vi "数据库查询.vi"() -> ()   [LabVIEW 2018]
uses:
  NPOI/net40/yt_ExcelLibrary.dll
  <vilib>/addons/database/Connection.llb/DB Tools Open Connec (String).vi
  <vilib>/addons/database/NI_Database_API.lvlib
  <vilib>/addons/_office/NI_ReportGenerationToolkit.lvlib
  <vilib>/Utility/NIReport.llb/Excel/NI_Excel.lvclass
  <vilib>/addons/_office/_exclsub.llb/font.ctl
  <vilib>/ptbypt/NI_PtbyPt.lvlib
  FreeMem.dll
  <vilib>/Utility/NIReport.llb/NI_report.lvclass
  <vilib>/Utility/NIReport.llb/Report Type.ctl
  <vilib>/Utility/NIReport.llb/NI_ReportGenerationCore.lvlib
  <vilib>/addons/_office/excel.llb/Excel Easy Table (str).vi
panel:
  out "错误输出":errorcluster
  out "数字(0-1)":dbl
  out "Elapsed Time (s)":dbl caption="已用时间(s)"
  out "2天时间到释放资源":bool caption="结束"
  in  "Main Tab":enum32{""}(tab)
  in  "时间范围OFF":bool
  in  "结束日期":timestamp
  in  "起始日期":timestamp
  in  "总成码OFF":bool
  in  "总成码":string
  in  "二维码OFF":bool
  in  "二维码":string
  in  "数据类型":u16(ring) items=["ALL", "Online", "Offline", "Rework"]
  in  "产品状态":u16(ring) items=["ALL", "OK", "NG"]
  in  "导出":bool
  in  "退出":bool
  in  "查询":bool
  in  "另存为":bool
  out "查询状态":string
  out "查询结果":i32(listbox)
  # "2020-04-14_17:08"
  # "历史数据查询"
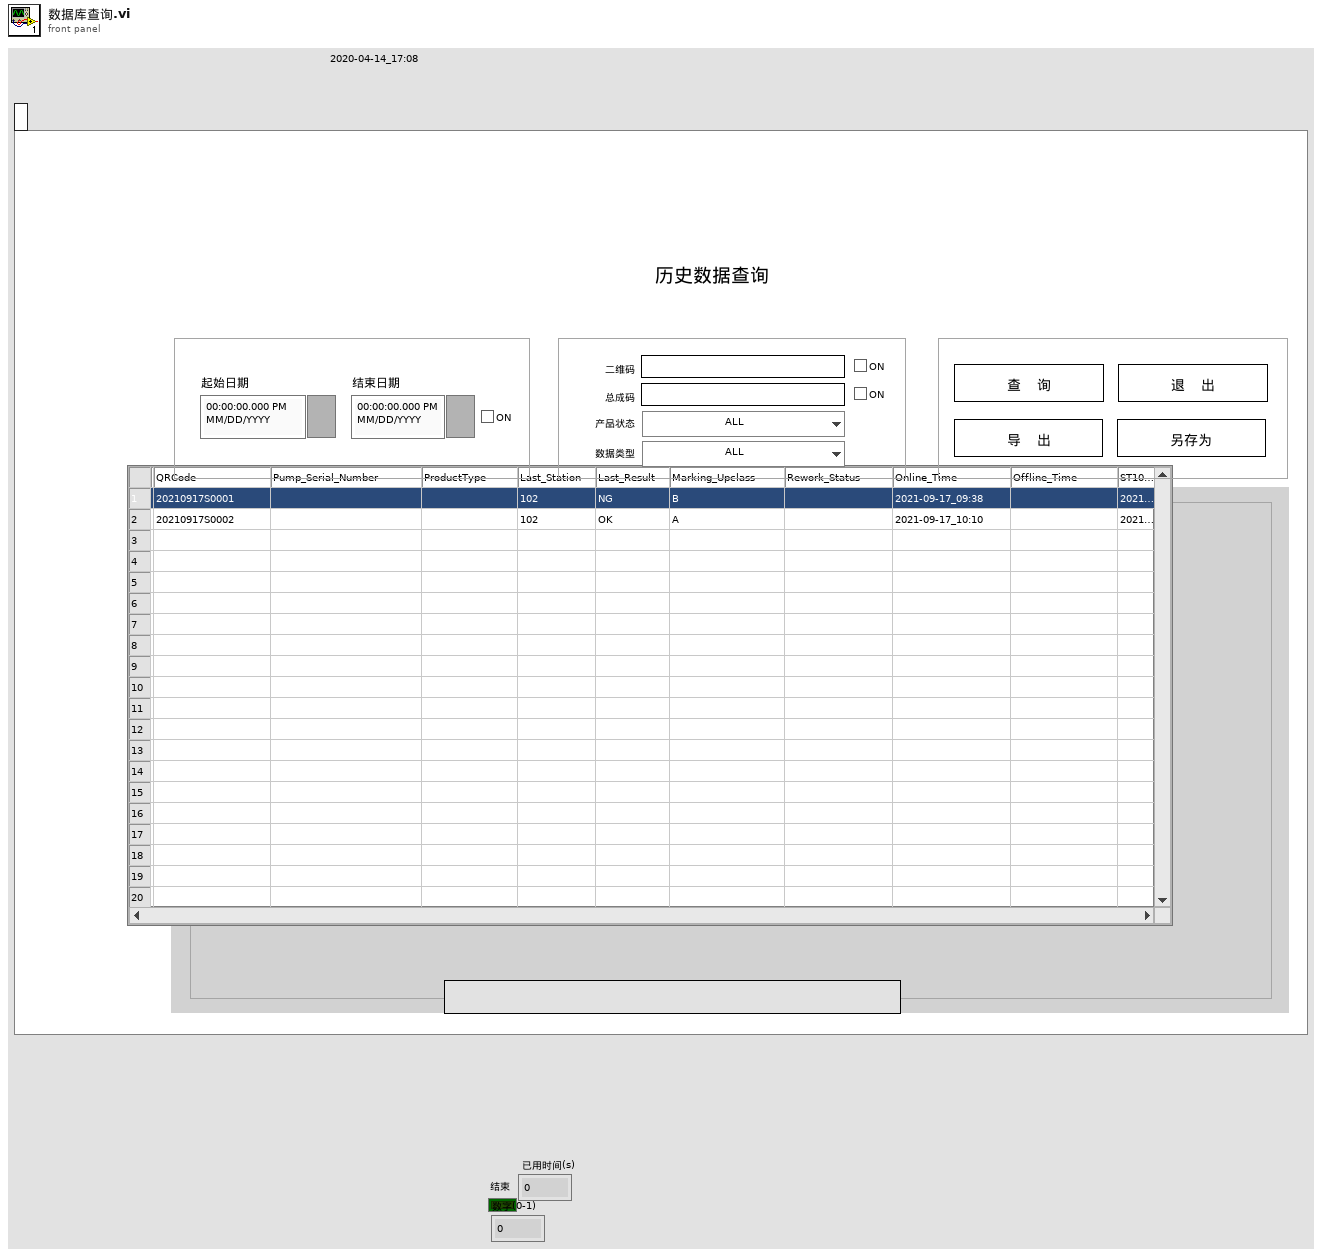
[diagram p1: front panel]
types:
  T1 = typedef "NI_ReportGenerationCore.lvlib/Report Type.ctl" = enum16{"HTML", "Word", "Excel"}
  T2 = typedef "NI_ReportGenerationToolkit.lvlib/font.ctl" = cluster{"font name":string, "font size":dbl, "bold":u16, "italic":u16, "underline":u16, "strike through":u16, "font color":u32}
  T3 = enum16{"maximized", "minimized", "normal", "no change"}
  T4 = enum32{"Invalid", "Standard", "Closed", "Hidden", "Minimized", "Maximized"}
  T5 = typedef "NI_Database_API.lvlib/Conn ObjectReference.ctl" = refnum<k1>
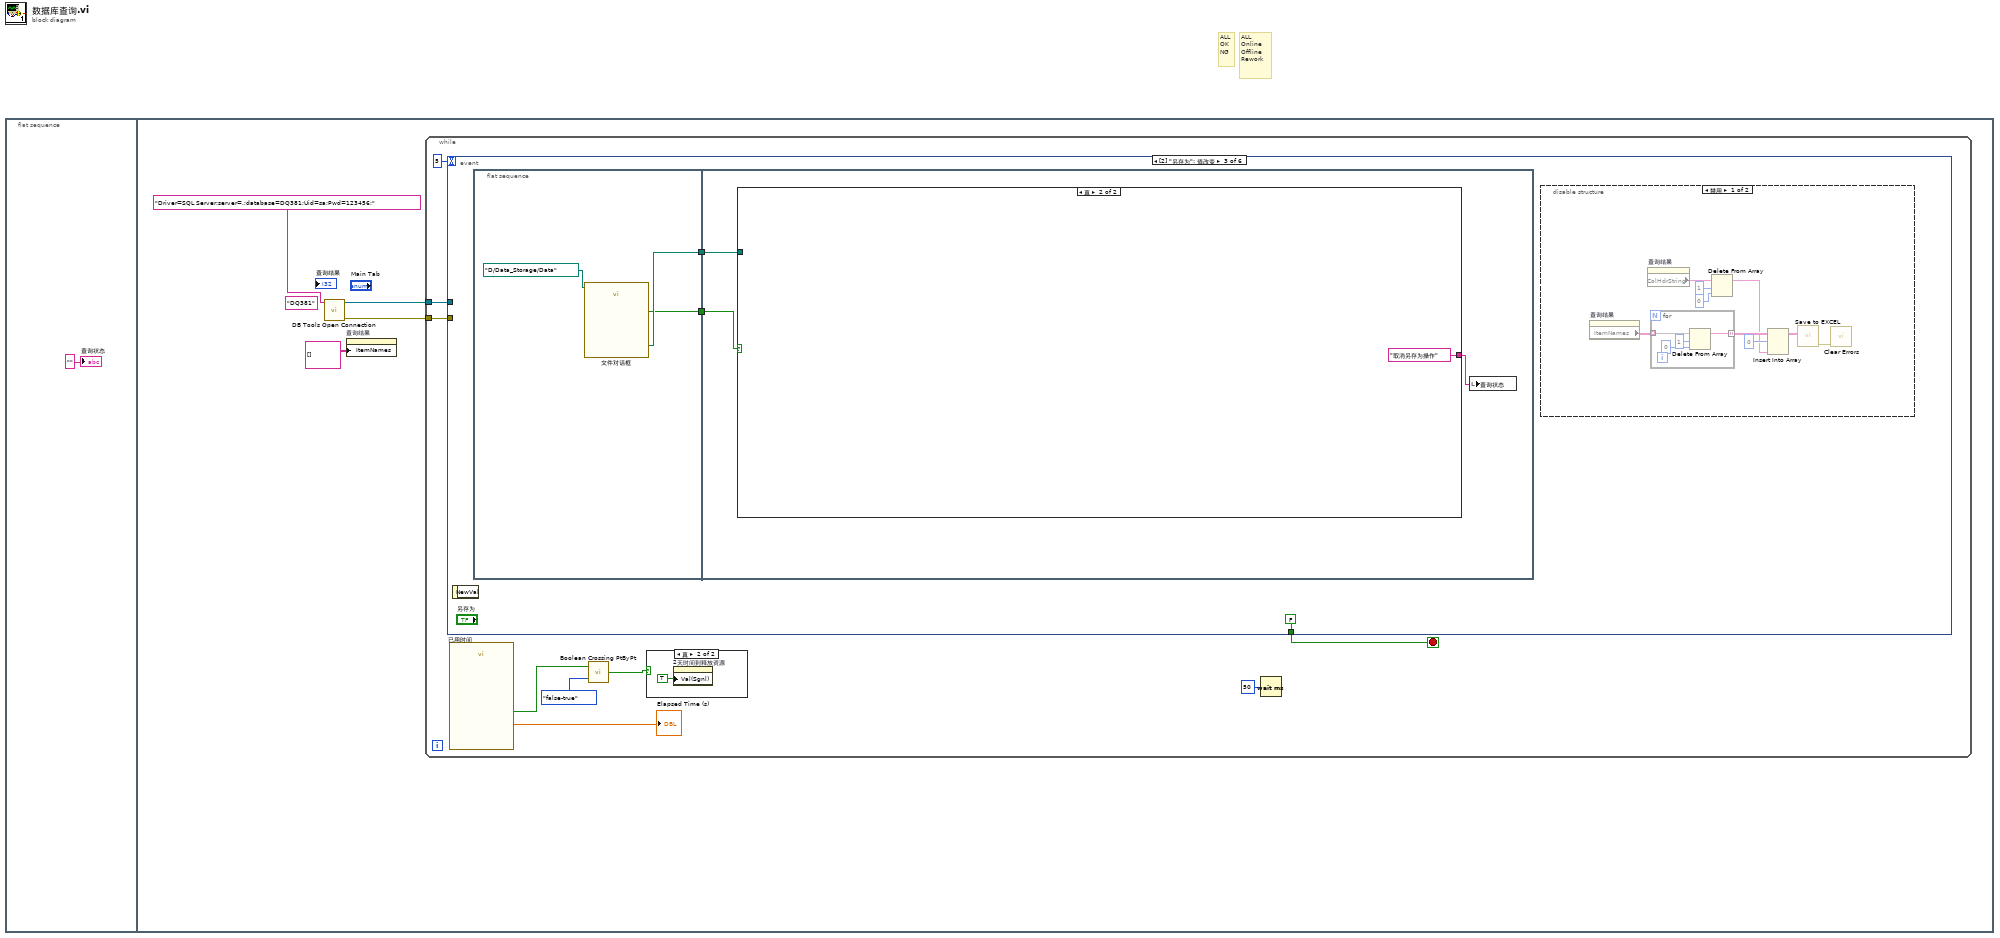
[diagram p0: block diagram]
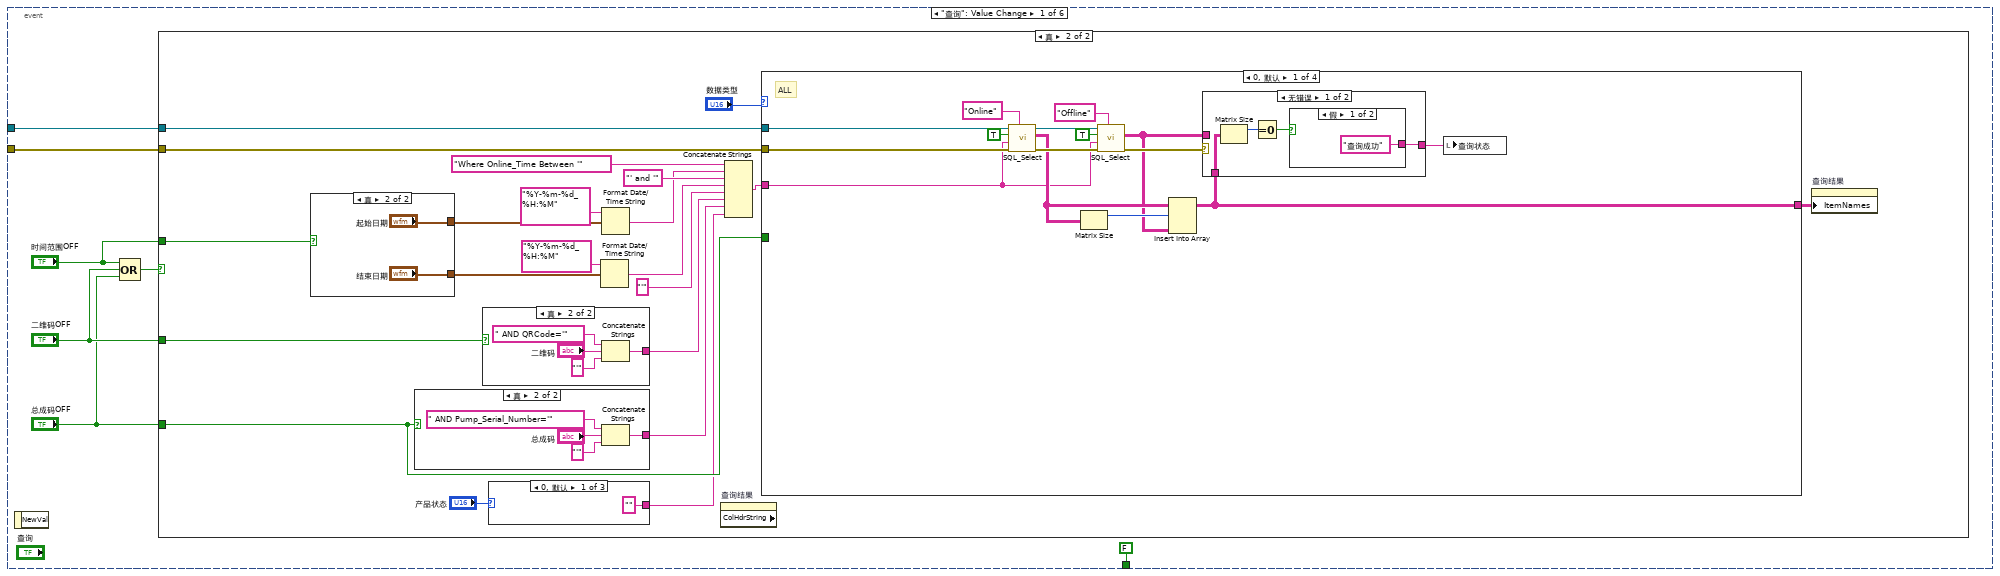
[diagram p3: hidden frame]
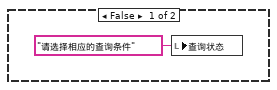
[diagram p4: hidden frame]
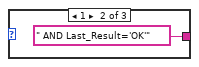
[diagram p5: hidden frame]
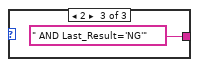
[diagram p6: hidden frame]
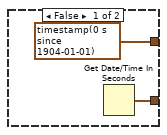
[diagram p7: hidden frame]
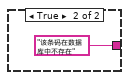
[diagram p8: hidden frame]
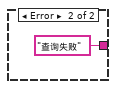
[diagram p9: hidden frame]
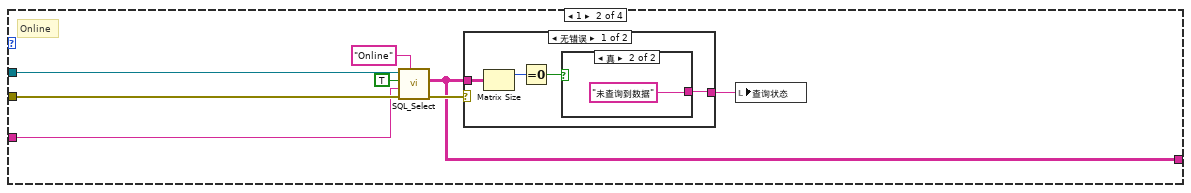
[diagram p10: hidden frame]
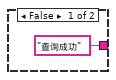
[diagram p11: hidden frame]
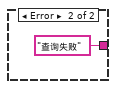
[diagram p12: hidden frame]
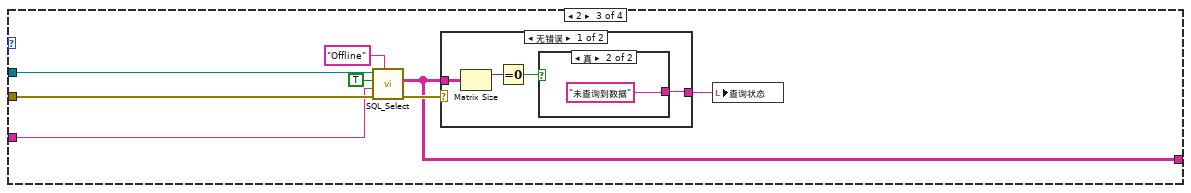
[diagram p13: hidden frame]
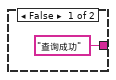
[diagram p14: hidden frame]
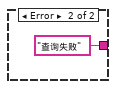
[diagram p15: hidden frame]
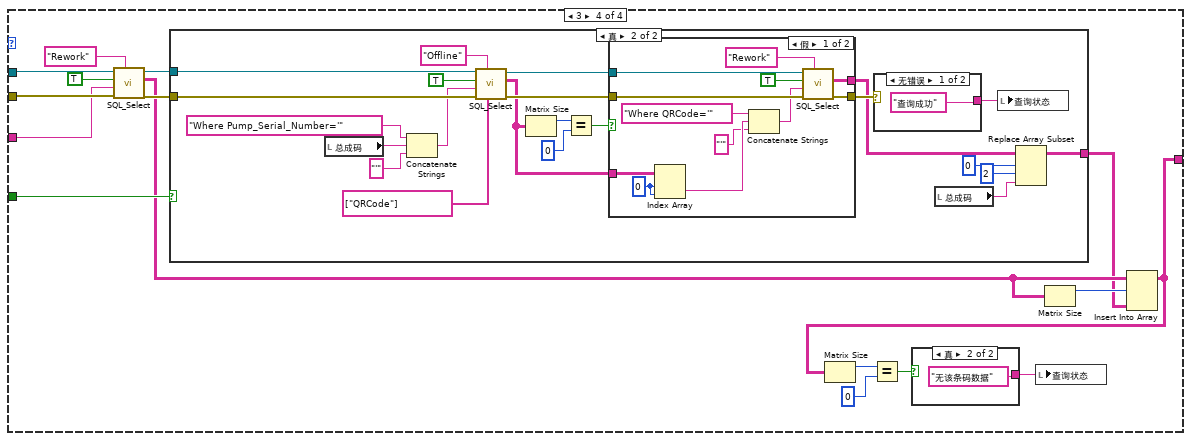
[diagram p16: hidden frame]
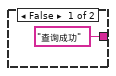
[diagram p17: hidden frame]
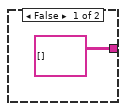
[diagram p18: hidden frame]
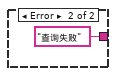
[diagram p19: hidden frame]
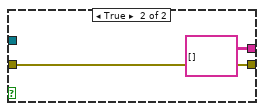
[diagram p20: hidden frame]
diagram:
  # "ALL\nOK\nNG"
  # "ALL\nOnline\nOffline\nRework"
  n1 = flat-sequence {
    frame #0 {
      "查询状态" <- "" ("查询状态")
    }
    frame #1 {
      (unwired) "DQ381"
      n2 = call-poly <vilib>:"DB Tools Open Connection.vi"("connection information"="Driver=SQL Server;server=.;database=DQ381;Uid=sa;Pwd=123456;") -> ("error out"=w4:errorcluster, "connection reference"=w5:T5)  [unwired: 7 in]
      n3 = property on="查询结果" class="MCListbox (严格)"("ItemNames"=string[][] [] ("项名")) -> ()  [unwired: 2 in, 2 out]
      n4 = while {
        tunnel: w5 -> [w14]
        tunnel: w4 -> [w13]
        stop <- w12 stop-if-true
        n5 = event shown="[2] \"另存为\": 值改变" {
          selector: _ -> [_ _ _ _ _ _]
          dyn-events: _ -> [_ _ _ _ _ _]
          timeout: 5 -> [_ _ _ _ _ _]
          tunnel: w14 -> [w22 _ _ _ w307 _]
          tunnel: w13 -> [w21 _ _ _ w306 _]
          tunnel: [FALSE ("NewVal") _ FALSE ("NewVal") _ w308 _] -> w12
          event "查询": Value Change {
            n6 = event-data() -> ()  [unwired: 1 in, 1 out]
            n7 = Compound Arithmetic op=OR("时间范围OFF", "二维码OFF", "总成码OFF") -> (w17:bool)
            n8 = case shown="真" w17 {
              tunnel: w22 -> [_ w44]
              tunnel: w21 -> [_ w43]
              tunnel: "二维码OFF" -> [_ w28]
              tunnel: "总成码OFF" -> [_ w27]
              tunnel: "时间范围OFF" -> [_ w26]
              frame False {
                n9 = local write "查询状态"("请选择相应的查询条件" ("查询状态")) -> ()
              }
              frame True {
                n10 = case shown="真" w26 {
                  tunnel: [timestamp(0 s since 1904-01-01) ("起始日期") "起始日期"] -> w39
                  tunnel: [w48 "结束日期"] -> w36
                  frame False {
                    n11 = Get Date/Time In Seconds() -> (seconds since 1Jan1904=w48:timestamp)
                  }
                  frame True {
                  }
                }
                n12 = case shown="真" w27 {
                  tunnel: ["" w163] -> w30
                  frame False {
                  }
                  frame True {
                    n13 = Concatenate Strings(" AND Pump_Serial_Number='" ("字符串"), "总成码", "'" ("字符串")) -> (w163:string)
                  }
                }
                n14 = case shown="真" w28 {
                  tunnel: ["" w167] -> w34
                  frame False {
                  }
                  frame True {
                    n15 = Concatenate Strings(" AND QRCode='" ("字符串"), "二维码", "'" ("字符串")) -> (w167:string)
                  }
                }
                n16 = case shown="0, 默认" "产品状态" {
                  tunnel: ["" " AND Last_Result='OK'" ("字符串") " AND Last_Result='NG'" ("字符串")] -> w24
                  frame 0, Default {
                  }
                  frame 1 {
                  }
                  frame 2 {
                  }
                }
                n17 = Format Date/Time String(time format string (%c)="%Y-%m-%d_%H:%M" ("时间格式字符串(%c)"), seconds (now)=w36) -> (date/time string=w35:string)  [unwired: 1 in]
                n18 = Format Date/Time String(time format string (%c)="%Y-%m-%d_%H:%M" ("时间格式字符串(%c)"), seconds (now)=w39) -> (date/time string=w38:string)  [unwired: 1 in]
                n19 = property on="查询结果" class="MCListbox (严格)" props=["ColHdrString"]() -> ()  [unwired: 2 in, 3 out]
                n20 = Concatenate Strings("Where Online_Time Between '" ("查询语句"), w38, "' and '" ("字符串"), w35, "'" ("字符串"), w34, w30, w24) -> (w33:string)
                n21 = case shown="0, 默认" "数据类型" {
                  tunnel: w44 -> [w66 w77 w92 w117]
                  tunnel: w43 -> [w65 w76 w91 w116]
                  tunnel: w33 -> [w56 w75 w90 w115]
                  tunnel: [w52 w74 w89 w108] -> w32
                  tunnel: w27 -> [_ _ _ w114]
                  frame 0, Default {
                    # "ALL"
                    n22 = call "SQL_Select.vi"("表名"="Online", "error in (no error)"=w65, "查询语句"=w56, "查询条件"=TRUE, "connection reference"=w66) -> ("error out"=w61:errorcluster, "数据"=w58:string[][], "connection reference out"=w60:T5)  [unwired: 4 in]
                    n23 = Matrix Size(0:w58) -> (1:w57:i32)  [unwired: 1 out]
                    n24 = call "SQL_Select.vi"("表名"="Offline", "error in (no error)"=w61, "查询语句"=w56, "查询条件"=TRUE, "connection reference"=w60) -> ("error out"=w55:errorcluster, "数据"=w53:string[][])  [unwired: 4 in, 1 out]
                    n25 = Insert Into Array(array=w58, index (row)=w57, new element=w53) -> (w52:string[][])  [unwired: 1 in]
                    n26 = case shown="无错误" w55 {
                      tunnel: [w68 "查询失败"] -> w54
                      tunnel: w53 -> [_ _]
                      tunnel: w52 -> [w67 _]
                      frame No Error {
                        n27 = Matrix Size(0:w67) -> (1:w70:i32)  [unwired: 1 out]
                        n28 = Equal To 0?(x=w70) -> (x = 0?=w69:bool)
                        n29 = case shown="假" w69 {
                          tunnel: ["查询成功" "该条码在数据库中不存在"] -> w68
                          frame False {
                          }
                          frame True {
                          }
                        }
                      }
                      frame Error {
                      }
                    }
                    n30 = local write "查询状态"(w54) -> ()
                  }
                  frame 1 {
                    # "Online"
                    n31 = call "SQL_Select.vi"("表名"="Online", "error in (no error)"=w76, "查询语句"=w75, "查询条件"=TRUE, "connection reference"=w77) -> ("error out"=w79:errorcluster, "数据"=w74:string[][])  [unwired: 4 in, 1 out]
                    n32 = case shown="无错误" w79 {
                      tunnel: [w83 "查询失败"] -> w78
                      tunnel: w74 -> [w82 _]
                      frame No Error {
                        n33 = Matrix Size(0:w82) -> (1:w85:i32)  [unwired: 1 out]
                        n34 = Equal To 0?(x=w85) -> (x = 0?=w84:bool)
                        n35 = case shown="真" w84 {
                          tunnel: ["查询成功" "未查询到数据"] -> w83
                          frame False {
                          }
                          frame True {
                          }
                        }
                      }
                      frame Error {
                      }
                    }
                    n36 = local write "查询状态"(w78) -> ()
                  }
                  frame 2 {
                    n37 = call "SQL_Select.vi"("表名"="Offline", "error in (no error)"=w91, "查询语句"=w90, "查询条件"=TRUE, "connection reference"=w92) -> ("error out"=w94:errorcluster, "数据"=w89:string[][])  [unwired: 4 in, 1 out]
                    n38 = case shown="无错误" w94 {
                      tunnel: [w98 "查询失败"] -> w93
                      tunnel: w89 -> [w97 _]
                      frame No Error {
                        n39 = Matrix Size(0:w97) -> (1:w100:i32)  [unwired: 1 out]
                        n40 = Equal To 0?(x=w100) -> (x = 0?=w99:bool)
                        n41 = case shown="真" w99 {
                          tunnel: ["查询成功" "未查询到数据"] -> w98
                          frame False {
                          }
                          frame True {
                          }
                        }
                      }
                      frame Error {
                      }
                    }
                    n42 = local write "查询状态"(w93) -> ()
                  }
                  frame 3 {
                    n43 = call "SQL_Select.vi"("表名"="Rework", "error in (no error)"=w116, "查询语句"=w115, "查询条件"=TRUE, "connection reference"=w117) -> ("error out"=w113:errorcluster, "数据"=w110:string[][], "connection reference out"=w112:T5)  [unwired: 4 in]
                    n44 = case shown="真" w114 {
                      tunnel: w113 -> [_ w144]
                      tunnel: w112 -> [_ w143]
                      tunnel: [string[][] [] ("数据") w123] -> w109
                      frame False {
                      }
                      frame True {
                        n45 = local read "总成码"() -> (w138:string)
                        n46 = Concatenate Strings("Where Pump_Serial_Number='" ("查询语句"), w138, "'" ("字符串")) -> (w137:string)
                        n47 = call "SQL_Select.vi"("要读取的列名"=string[] ["QRCode"], "表名"="Offline", "error in (no error)"=w144, "查询语句"=w137, "查询条件"=TRUE, "connection reference"=w143) -> ("error out"=w131:errorcluster, "数据"=w130:string[][], "connection reference out"=w132:T5)  [unwired: 3 in]
                        n48 = Matrix Size(0:w130) -> (1:w135:i32)  [unwired: 1 out]
                        n49 = Equal?(x=w135, y=0) -> (x = y?=w133:bool)
                        n50 = case shown="假" w133 {
                          tunnel: w132 -> [w158 _]
                          tunnel: w131 -> [w157 w160]
                          tunnel: [w154 string[][] [] ("数据")] -> w127
                          tunnel: [w153 w160] -> w128
                          tunnel: w130 -> [w150 _]
                          frame False {
                            w149 = 0 ("索引 (行)")
                            n51 = Index Array(array=w150, index (row)=w149, index (col)=w149) -> (element=w148:string)
                            n52 = Concatenate Strings("Where QRCode='" ("查询语句"), w148, "'" ("字符串")) -> (w152:string)
                            n53 = call "SQL_Select.vi"("表名"="Rework", "error in (no error)"=w157, "查询语句"=w152, "查询条件"=TRUE, "connection reference"=w158) -> ("error out"=w153:errorcluster, "数据"=w154:string[][])  [unwired: 4 in, 1 out]
                          }
                          frame True {
                          }
                        }
                        n54 = case shown="无错误" w128 {
                          tunnel: ["查询成功" "查询失败"] -> w129
                          frame No Error {
                          }
                          frame Error {
                          }
                        }
                        n55 = local read "总成码"() -> (w124:string)
                        n56 = local write "查询状态"(w129) -> ()
                        n57 = Replace Array Subset(array=w127, new element=w124, index (row)=0 ("索引 (行)"), index (col)=2 ("禁用的索引 (列)")) -> (w123:string[][])
                      }
                    }
                    n58 = Matrix Size(0:w110) -> (1:w111:i32)  [unwired: 1 out]
                    n59 = Insert Into Array(array=w110, index (row)=w111, new element=w109) -> (w108:string[][])  [unwired: 1 in]
                    n60 = Matrix Size(0:w108) -> (1:w107:i32)  [unwired: 1 out]
                    n61 = Equal?(x=w107, y=0) -> (x = y?=w104:bool)
                    n62 = case shown="真" w104 {
                      tunnel: ["查询成功" "无该条码数据"] -> w105
                      frame False {
                      }
                      frame True {
                      }
                    }
                    n63 = local write "查询状态"(w105) -> ()
                  }
                }
                n64 = property on="查询结果" class="MCListbox (严格)"("ItemNames"=w32) -> ()  [unwired: 2 in, 2 out]
              }
            }
          }
          event Timeout {
            n65 = event-data() -> ()  [unwired: 1 in, 3 out]
          }
          event "另存为": Value Change {
            n66 = event-data() -> ()  [unwired: 1 in, 1 out]
            n67 = flat-sequence {
              tunnel: [w175] -> w172
              tunnel: [w174] -> w171
              tunnel: w172 -> [w178]
              tunnel: w171 -> [w177]
              frame #0 {
                n68 = call "文件对话框"("start path"=path "D:/Data_Storage/Data" ("文件路径（使用对话框）")) -> ("selected path"=w175:path, "cancelled"=w174:bool)  [unwired: 11 in, 2 out]
              }
              frame #1 {
                n69 = case shown="真" w177 {
                  tunnel: [w181 "取消另存为操作"] -> w179
                  tunnel: w178 -> [w180 _]
                  frame False {
                    n70 = disable-structure shown="启用" {
                      disable-tunnel: [w203 string[][] [["1", "2", "3", "4", "5", "6"], ["9", "8", "7", "6", "5", "4"]]] -> w185
                      frame Enabled {
                        n71 = property on="查询结果" class="MCListbox (严格)"() -> ("ItemNames"=w206:string[][])  [unwired: 2 in, 2 out]
                        n72 = property on="查询结果" class="MCListbox (严格)"() -> ("ColHdrString"=w209:string[])  [unwired: 2 in, 2 out]
                        n73 = Delete From Array(array=w209, length=1 ("长度"), index=0 ("索引")) -> (array with subset deleted=w202:string[])  [unwired: 1 out]
                        n74 = for {
                          tunnel: w206 -> [w213] mode=indexing
                          tunnel: [w210] -> w204 mode=indexing
                          n75 = Delete From Array(array=w213, length=1 ("长度"), index=0 ("索引")) -> (array with subset deleted=w210:string[])  [unwired: 1 out]
                        }
                        n76 = Insert Into Array(array=w204, index (row)=0 ("索引"), new element=w202) -> (w203:string[][])  [unwired: 1 in]
                      }
                      frame Disabled {
                      }
                    }
                    n77 = Format Date/Time String(time format string (%c)="%Y%m%d%H%M%S" ("时间格式字符串(%c)")) -> (date/time string=w200:string)  [unwired: 2 in]
                    n78 = Concatenate Strings(w200, ".xlsx" ("字符串")) -> (w198:string)
                    n79 = Build Path(base path=w180, name or relative path=w198) -> (appended path=w196:path)
                    n80 = Path To String(path=w196) -> (string=w193:string)
                    n81 = call <vilib>:"To .NET Object.vi"("anything"=w185) -> (".NET object"=w184:refnum<k24>)  [unwired: 1 in, 1 out]
                    n82 = constructor class="ExcelHelper"("strFileName"=w193) -> (reference out=w195:refnum<k24>, error out=w194:errorcluster)  [unwired: 3 in, 2 out]
                    n83 = invoke on="调用节点" class="ExcelHelper" method="ObjectToExcel"(reference=w195, error in=w194, "obj"=w184, "sheetName"="ExportData", "isColumnWritten"=TRUE, "isConversionDouble"=FALSE, "isAddToOriginal"=FALSE) -> (reference out=w183:refnum<k24>, error out=w182:errorcluster, "strErr"=w189:string)  [unwired: 2 in, 6 out]
                    n84 = Equal?(x=w189, y="") -> (x = y?=w187:bool)
                    n85 = Close Reference(reference=w183, error in (no error)=w182) -> ()  [unwired: 1 out]
                    n86 = case shown="假" w187 {
                      tunnel: [w218 errorcluster {"status"=FALSE, "code"=0, "source"=""} ("error IO")] -> w197
                      tunnel: w189 -> [w215 _]
                      frame False {
                        n87 = Bundle By Name(cluster=errorcluster {"status"=FALSE, "code"=0, "source"=""} ("error IO"), "status"=TRUE, "code"=0, "source"=w215) -> (w218:errorcluster)
                      }
                      frame True {
                      }
                    }
                    n88 = case shown="错误" w197 {
                      tunnel: ["导出成功" "导出失败"] -> w181
                      frame No Error {
                      }
                      frame Error {
                      }
                    }
                  }
                  frame True {
                  }
                }
                n89 = local write "查询状态"(w179) -> ()
              }
            }
            n90 = disable-structure shown="禁用" {
              frame Disabled {
                n91 = property on="查询结果" class="MCListbox (严格)"() -> ("ItemNames"=w229:string[][])  [unwired: 2 in, 2 out]
                n92 = property on="查询结果" class="MCListbox (严格)"() -> ("ColHdrString"=w232:string[])  [unwired: 2 in, 2 out]
                n93 = for {
                  tunnel: w229 -> [w236] mode=indexing
                  tunnel: [w233] -> w227 mode=indexing
                  n94 = Delete From Array(array=w236, length=1 ("长度"), index=0 ("索引")) -> (array with subset deleted=w233:string[])  [unwired: 1 out]
                }
                n95 = Delete From Array(array=w232, length=1 ("长度"), index=0 ("索引")) -> (array with subset deleted=w226:string[])  [unwired: 1 out]
                n96 = Insert Into Array(array=w227, index (row)=0 ("索引"), new element=w226) -> (w225:string[][])  [unwired: 1 in]
                n97 = call "Save to EXCEL.vi"("text data"=w225) -> ("error out"=w224:errorcluster)  [unwired: 10 in]
                n98 = call <vilib>:"Clear Errors.vi"("error in (no error)"=w224) -> ()  [unwired: 5 in, 2 out]
              }
              frame Enabled {
              }
            }
          }
          event "导出": Value Change {
            n99 = event-data() -> ()  [unwired: 1 in, 3 out]
            n100 = disable-structure shown="启用" {
              disable-tunnel: [w264 string[][] [["1", "2", "3", "4", "5", "6"], ["9", "8", "7", "6", "5", "4"]]] -> w240
              frame Enabled {
                n101 = property on="查询结果" class="MCListbox (严格)"() -> ("ItemNames"=w267:string[][])  [unwired: 2 in, 2 out]
                n102 = property on="查询结果" class="MCListbox (严格)"() -> ("ColHdrString"=w270:string[])  [unwired: 2 in, 2 out]
                n103 = Delete From Array(array=w270, length=1 ("长度"), index=0 ("索引")) -> (array with subset deleted=w263:string[])  [unwired: 1 out]
                n104 = for {
                  tunnel: w267 -> [w274] mode=indexing
                  tunnel: [w271] -> w265 mode=indexing
                  n105 = Delete From Array(array=w274, length=1 ("长度"), index=0 ("索引")) -> (array with subset deleted=w271:string[])  [unwired: 1 out]
                }
                n106 = Insert Into Array(array=w265, index (row)=0 ("索引"), new element=w263) -> (w264:string[][])  [unwired: 1 in]
              }
              frame Disabled {
              }
            }
            n107 = call <vilib>:"Check if File or Folder Exists.vi"("path"=path "D:/Data_Storage/Data" ("文件路径（使用对话框）")) -> ("error out"=w259:errorcluster, "file or folder exists?"=w261:bool, "dup path"=w260:path)  [unwired: 8 in]
            n108 = Format Date/Time String(time format string (%c)="%Y%m%d%H%M%S" ("时间格式字符串(%c)")) -> (date/time string=w257:string)  [unwired: 2 in]
            n109 = case shown="假" w261 {
              tunnel: w260 -> [w301 w303]
              tunnel: [w300 w303] -> w255
              tunnel: w259 -> [w299 w302]
              tunnel: [w298 w302] -> _
              frame False {
                n110 = Create Folder(path (use dialog)=w301, error in=w299) -> (created path=w300:path, error out=w298:errorcluster)  [unwired: 1 in, 1 out]
              }
              frame True {
              }
            }
            n111 = Concatenate Strings(w257, ".xlsx" ("字符串")) -> (w254:string)
            n112 = Build Path(base path=w255, name or relative path=w254) -> (appended path=w251:path)
            n113 = Path To String(path=w251) -> (string=w248:string)
            n114 = call <vilib>:"To .NET Object.vi"("anything"=w240) -> (".NET object"=w239:refnum<k24>)  [unwired: 1 in, 1 out]
            n115 = constructor class="ExcelHelper"("strFileName"=w248) -> (reference out=w250:refnum<k24>, error out=w249:errorcluster)  [unwired: 3 in, 2 out]
            n116 = invoke on="调用节点" class="ExcelHelper" method="ObjectToExcel"(reference=w250, error in=w249, "obj"=w239, "sheetName"="ExportData", "isColumnWritten"=TRUE, "isConversionDouble"=FALSE, "isAddToOriginal"=FALSE) -> (reference out=w238:refnum<k24>, error out=w237:errorcluster, "strErr"=w244:string)  [unwired: 2 in, 6 out]
            n117 = Equal?(x=w244, y="") -> (x = y?=w242:bool)
            n118 = Close Reference(reference=w238, error in (no error)=w237) -> ()  [unwired: 1 out]
            n119 = case shown="假" w242 {
              tunnel: [w279 errorcluster {"status"=FALSE, "code"=0, "source"=""} ("error IO")] -> w252
              tunnel: w244 -> [w276 _]
              frame False {
                n120 = Bundle By Name(cluster=errorcluster {"status"=FALSE, "code"=0, "source"=""} ("error IO"), "status"=TRUE, "code"=0, "source"=w276) -> (w279:errorcluster)
              }
              frame True {
              }
            }
            n121 = case shown="错误" w252 {
              tunnel: ["导出成功" "导出失败"] -> w253
              frame No Error {
              }
              frame Error {
              }
            }
            n122 = local write "查询状态"(w253) -> ()
            n123 = disable-structure shown="禁用" {
              frame Disabled {
                (unwired) path "D:/Model/EXCEL.xlsx" ("template (empty)")
                w294 = 1 items=["left", "center", "right"] ("horizontal alignment (left)")
                n124 = call <vilib>:"Create Report.vi"("window state (normal)"=T3."no change", "report type"=Report_Type."Excel") -> ("report out"=w283:refnum<class "NI_report.lvclass">, "error out"=w282:errorcluster)  [unwired: 12 in]
                n125 = call-poly <vilib>:"Excel Easy Table.vi"("report in"=w283, "font"=T2 {"font name"="", "font size"=12.0, "bold"=0, "italic"=0, "underline"=0, "strike through"=0, "font color"=16777216}, "start (0, 0)"=cluster{"row":i32, "column":i32} {"row"=0, "column"=0}, "error in (no error)"=w282) -> ("report out"=w292:refnum<class "NI_report.lvclass">, "error out"=w293:errorcluster)  [unwired: 7 in, 3 out]
                n126 = call <vilib>:"Excel Set Cell Alignment.vi"("report in"=w292, "horizontal alignment (left)"=w294, "error in (no error)"=w293) -> ("report out"=w287:refnum<class "NI_report.lvclass">, "error out"=w290:errorcluster)  [unwired: 11 in]
                n127 = call-dynamic "Save Report to File.vi"("report in"=w287, "error in (no error)"=w290) -> ("report out"=w288:refnum<class "NI_report.lvclass">, "error out"=w289:errorcluster)  [unwired: 12 in]
                n128 = call-dynamic "Dispose Report.vi"("report in"=w288, "error in (no error)"=w289) -> ("error out"=w286:errorcluster)  [unwired: 13 in]
                n129 = call <vilib>:"Clear Errors.vi"("error in (no error)"=w286) -> ()  [unwired: 5 in, 2 out]
              }
              frame Enabled {
              }
            }
          }
          event "退出": Value Change {
            n130 = event-data() -> ("NewVal"=w308:bool)  [unwired: 1 in]
            n131 = call <vilib>:"DB Tools Close Connection.vi"("error in (no error)"=w306, "connection reference"=w307) -> ()  [unwired: 5 in, 1 out]
            n132 = control-ref of="本VI"() -> (w305:refnum<vi>)
            n133 = property class="VI"(reference=w305, "FP.State"=T4."Closed" ("前面板窗口:状态")) -> ()  [unwired: 1 in, 2 out]
          }
          event "2天时间到释放资源": Value Change {
            n134 = event-data() -> ()  [unwired: 1 in, 3 out]
            n135 = Random Number (0-1)() -> (number: 0 to 1=→"数字(0-1)":dbl)
            n136 = dll-call lib="PTH2abs E$èå·åæ³°ç§æè¡ä»½æéå¬å¸é¡¹ç®éº¦æ ¼çº³ç¨åºDQ381DQ501æ¹é -YT20-031381381-LV2018Project-20211216ProjectFreeMem.dll" fn="FreeMem"() -> (error out=→"错误输出":errorcluster)  [unwired: 4 in, 1 out]
          }
        }
        n137 = call "已用时间"() -> ("Elapsed Time (s)"=→"Elapsed Time (s)":dbl, "Time has Elapsed"=w8:bool)  [unwired: 12 in, 6 out]
        n138 = call <vilib>:"Boolean Crossing PtByPt.vi"("direction"=enum16{"either", "false-true", "true-false"}."false-true", "input"=w8) -> ("crossing"=w7:bool)  [unwired: 1 in]
        n139 = case shown="真" w7 {
          frame False {
          }
          frame True {
            n140 = property on="2天时间到释放资源" class="Bool (严格)"("Val(Sgnl)"=TRUE ("值(信号)")) -> ()  [unwired: 2 in, 2 out]
          }
        }
        n141 = Wait (ms)(milliseconds to wait=u32 50 ("等待时间（毫秒）")) -> ()  [unwired: 1 out]
      }
    }
  }
